vi "Sim Phone.vi"() -> ()   [LabVIEW 2019]
doc: "This vi demonstrates how to output waveform using SO Waveform Scan vi.\nIt also reveals the basic principle of telephone tone generation -- every tone consists of two sine waves of different frequency."
uses:
  <vilib>/sound/lvsound.llb/Sound Format.ctl
  <vilib>/express/express analysis/Spectral/Block/exnSpectralBlock spectral measurements RMS poly.vi
  <vilib>/express/express analysis/Spectral/Block/exnSpectralBlock spectral measurements RMS WFM.vi
  <vilib>/express/express analysis/Spectral/XNode/ExpressSpectralMeasurementsBlockNode.xnode
  <vilib>/measure/NI_MAPro.lvlib
panel:
  out "FFT":cluster{"f0":dbl, "df":dbl, "magnitude":dbl[]}(graph)={"f0"=0.0, "df"=1.0, "magnitude"=array[22050 elements]}
  out "Waveform Graph":waveform(dbl)(graph)={"t0"=timestamp(0 s since 1904-01-01), "dt"=2.2675736961451248e-05, "Y"=array[44100 elements]}
  in  "volume":dbl(slide)=0.6095238095238096 scale=0.0..1.0 scale format="%0.1f"
  in  "keys":T1
  in  "stop":bool
  # "Run the VI. Press the keypad to generate different tones\nand adjust volume by moving the slider.\n(Based on old SimPhone example)"
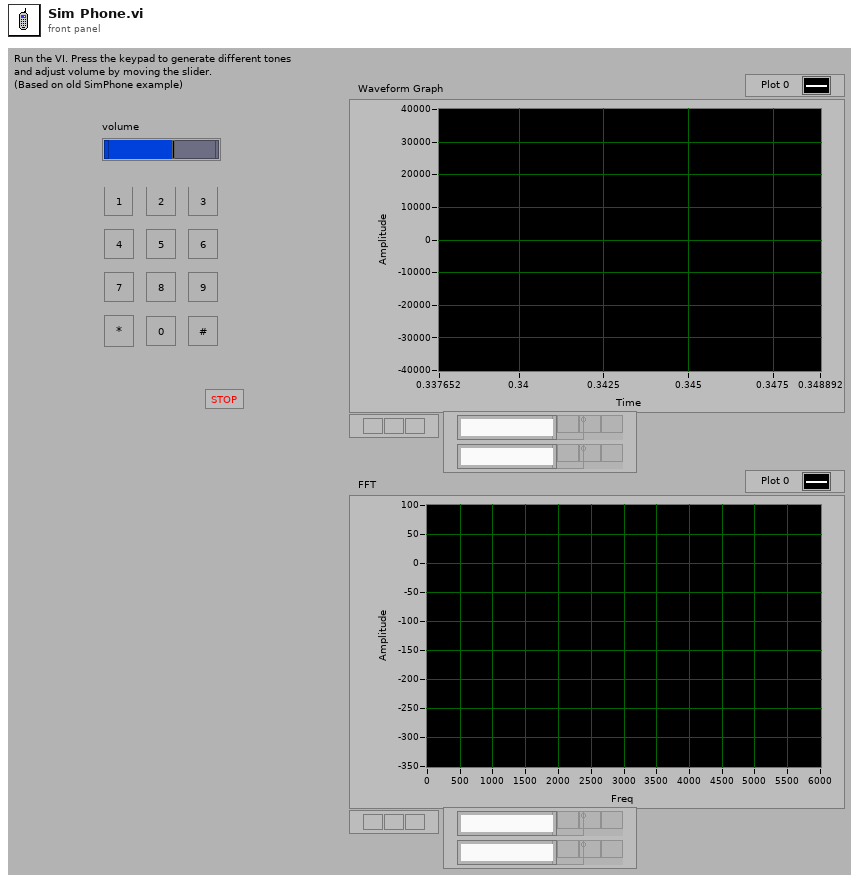
[diagram p1: front panel]
types:
  T1 = cluster{bool, bool, bool, bool, bool, bool, bool, bool, bool, bool, bool, bool}
  T2 = typedef "Sound Format.ctl" = cluster{"sound quality":enum16{"mono", "stereo"}, "rate":enum16{"11025", "22050", "44100", "8000"}, "bits per sample":enum16{"8 bit", "16 bit"}}
  T3 = cluster{"averaging mode":u16, "weighting mode":u16, "number of averages":u32}
  T4 = cluster{"dB On (F)":bool, "unwrap phase (F)":bool, "convert to degree (F)":bool}
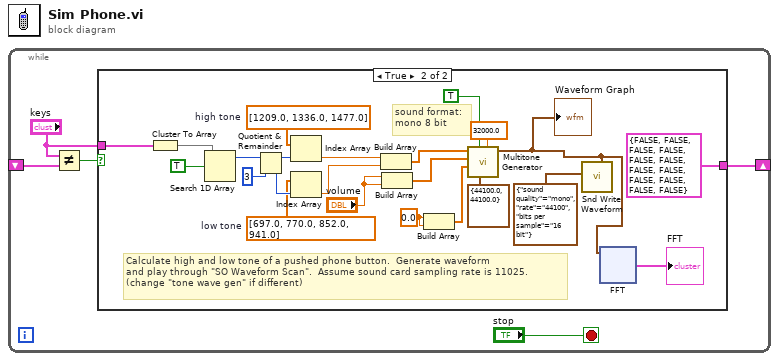
[diagram p0: block diagram]
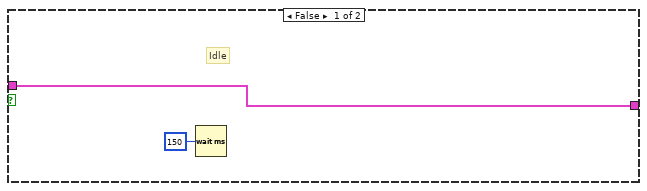
[diagram p2: hidden frame]
diagram:
  n1 = while {
    shift-left: _ -> [w2]
    shift-right: [w4] -> _
    stop <- "stop" stop-if-true
    n2 = Not Equal?(x="keys", y=w2) -> (x != y?=w5:bool)
    n3 = case shown="True" w5 {
      tunnel: "keys" -> [w7 w22]
      tunnel: [w7 T1 {FALSE, FALSE, FALSE, FALSE, FALSE, FALSE, FALSE, FALSE, FALSE, FALSE, FALSE, FALSE}] -> w4
      frame False {
        # "Idle"
        n4 = Wait (ms)(milliseconds to wait=u32 150) -> ()  [unwired: 1 out]
      }
      frame True {
        w12 = 0.0 ("element")
        w23 = dbl[] [1209.0, 1336.0, 1477.0]  # high tone
        w24 = dbl[] [697.0, 770.0, 852.0, 941.0]  # low tone
        # "sound format:\nmono 8 bit"
        # "Calculate high and low tone of a pushed phone button.  Generate waveform\nand play through \"SO Waveform Scan\".  Assume sound card sampling rate is 11025.\n(change \"tone wave gen\" if different)"
        n5 = Cluster To Array(cluster=w22) -> (array=w30:bool[])
        n6 = Search 1D Array(1D array=w30, element=TRUE) -> (index of element=w28:i32)  [unwired: 1 in]
        n7 = Quotient & Remainder(x=w28, y=3) -> (x-y*floor(x/y)=w26:i32, floor(x/y)=w25:i32)
        n8 = Index Array(array=w23, index=w26) -> (element=w15:dbl)
        n9 = Index Array(array=w24, index=w25) -> (element=w19:dbl)
        n10 = Build Array(w15, w19) -> (w18:dbl[])
        n11 = Build Array("volume", "volume") -> (w20:dbl[])
        n12 = Build Array(w12, w12) -> (w16:dbl[])
        n13 = call <vilib>:"Multitone Generator.vi"("amplitude"=32000.0, "sampling info"=cluster{"Fs":dbl, "#s":dbl} {"Fs"=44100.0, "#s"=44100.0}, "reset signal"=TRUE, "tone phases"=w16, "tone amplitudes"=w20, "tone frequencies"=w18) -> ("signal out"=w8:waveform(dbl))  [unwired: 2 in, 3 out]
        "Waveform Graph" <- w8
        n14 = call <vilib>:"Snd Write Waveform.vi"("mono 16-bit"=w8, "sound format"=T2 {"sound quality"=enum."mono", "rate"=enum."44100", "bits per sample"=enum."16 bit"}) -> ()  [unwired: 9 in, 1 out]
        n15 = xnode "FFT"("Signals"=w8) -> ("FFT - (RMS)"=→"FFT":cluster{"f0":dbl, "df":dbl, "magnitude":dbl[]})  [unwired: 1 in, 2 out]
      }
    }
  }
